vi "ReadLockin_ETH_2median.vi"(0 "Delay (ms)":u32, 1 "Lockin Address":string="1:8", 2 "Integration (ms)":u32=1000, 3 "data storage rate (Hz)":u16(ring)=7 items=[".0625 ", "0.125 ", "0.250 ", "0.500 ", "1 ", "2 ", "4", "8 ", "16 ", "32 ", "64 ", "128", "256", "512"], 5 "error in":errorcluster) -> (6 "R":dbl=0.0024531641755826043, 7 "Theta (radians)":dbl=2.561846938936039, 8 "error out":errorcluster)   [LabVIEW 2023]
uses:
  <vilib>/Analysis/NI_AALBase.lvlib
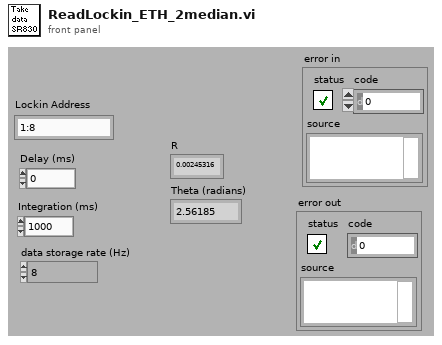
[diagram p1: front panel]
types:
  T1 = cluster{"error":bool, "code":i32, "source":string}
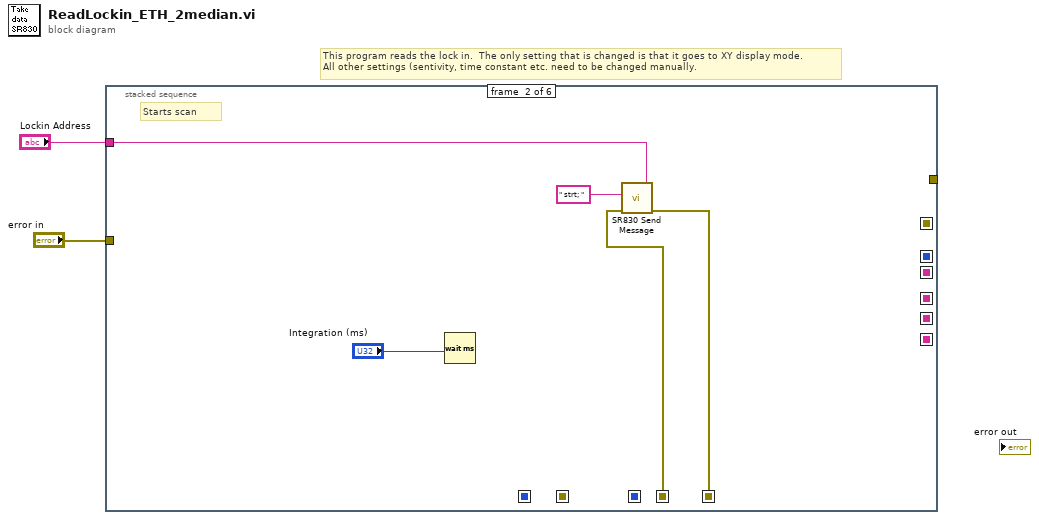
[diagram p0: block diagram]
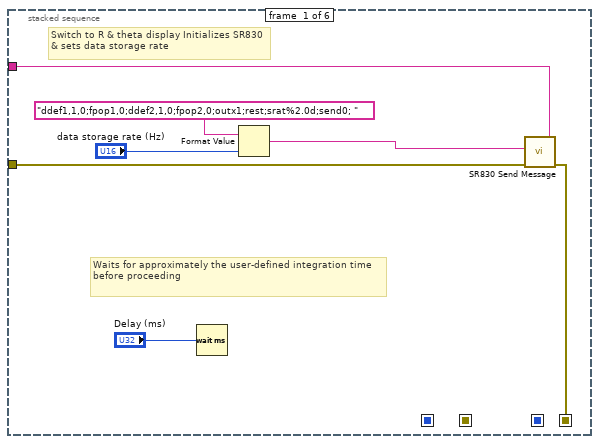
[diagram p2: hidden frame]
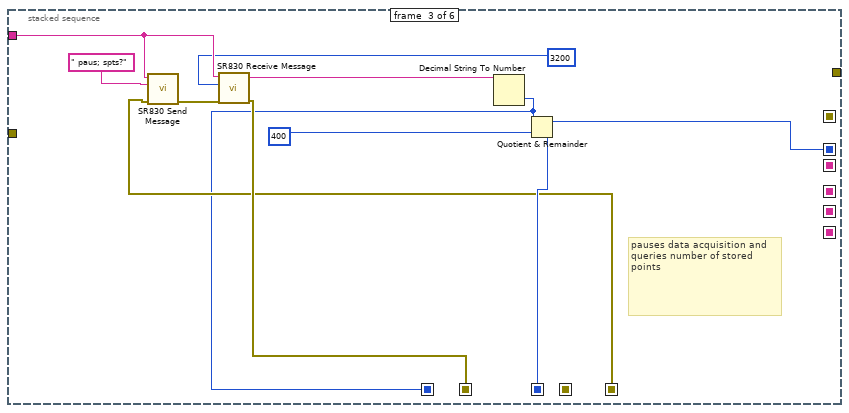
[diagram p3: hidden frame]
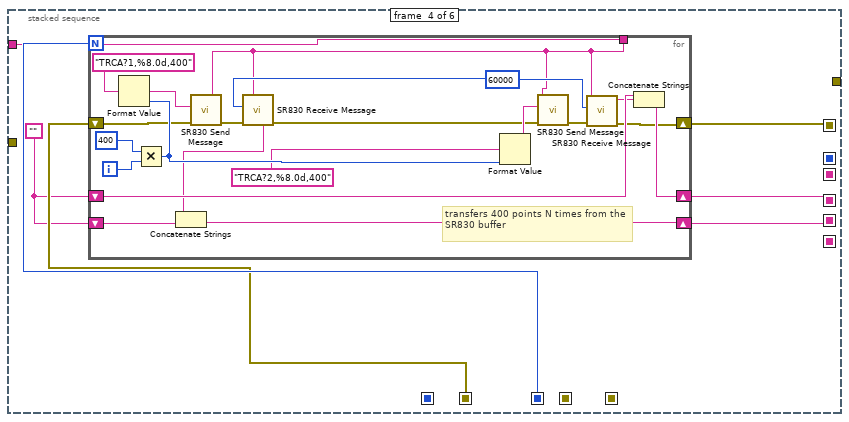
[diagram p4: hidden frame]
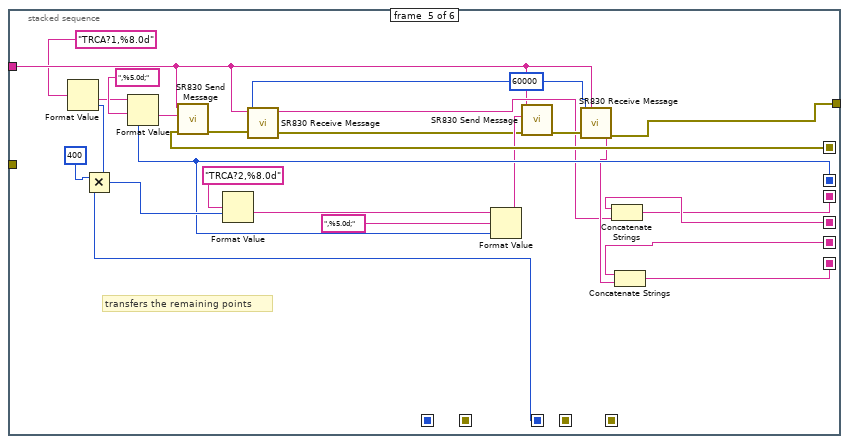
[diagram p5: hidden frame]
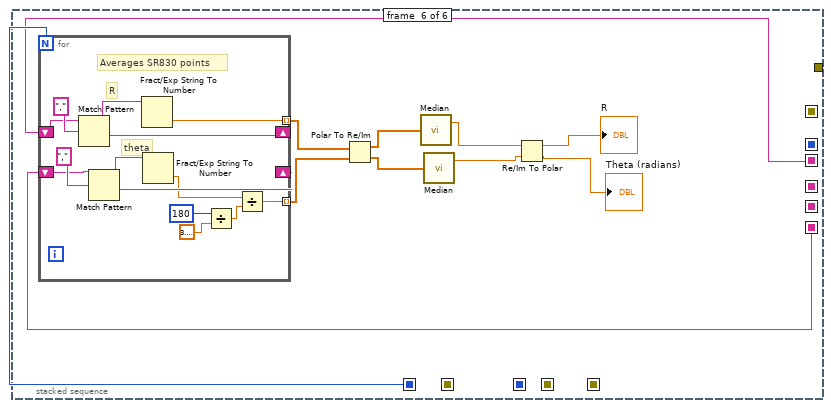
[diagram p6: hidden frame]
diagram:
  # "This program reads the lock in.  The only setting that is changed is that it goes to XY display mode.\nAll other settings (sentivity, time constant etc. need to be changed manually."
  n1 = stacked-sequence {
    seq-local: [w8 _ _ _ _ _] -> [_ w13 _ _ _ _]
    seq-local: [_ _ w24 _ _ _] -> [_ _ _ _ w74 _]
    seq-local: [_ _ w23 _ _ _] -> [_ _ _ w32 w76 _]
    seq-local: [_ _ w17 _ _ _] -> [_ _ _ w30 _ _]
    seq-local: [_ _ _ w28 _ _] -> [_ _ _ _ w71 _]
    seq-local: [_ _ _ w27 _ _] -> [_ _ _ _ w73 _]
    seq-local: [_ _ _ w26 _ _] -> [_ _ _ _ w72 _]
    seq-local: [_ _ w15 _ _ _] -> [_ _ _ _ _ w88]
    seq-local: [_ _ _ _ w54 _] -> [_ _ _ _ _ w86]
    seq-local: [_ _ _ _ w53 _] -> [_ _ _ _ _ w87]
    seq-local: [_ w12 _ _ _ _] -> [_ _ w16 _ _ _]
    tunnel: "error in" -> [w9 _ _ _ _ _]
    tunnel: "Lockin Address" -> [w7 w14 w21 w31 w64 _]
    tunnel: [_ _ _ _ w68 _] -> _
    frame #0 {
      # "Waits for approximately the user-defined integration time before proceeding"
      # "Switch to R & theta display Initializes SR830 & sets data storage rate"
      n2 = Wait (ms)(milliseconds to wait="Delay (ms)") -> ()  [unwired: 1 out]
      n3 = Format Value(format string="ddef1,1,0;fpop1,0;ddef2,1,0;fpop2,0;outx1;rest;srat%2.0d;send0; ", value (0)="data storage rate (Hz)") -> (output string=w4:string)  [unwired: 1 in]
      n4 = call "SR830 Send Message.vi"("address string"=w7, "write buffer"=w4, "error in"=w9) -> ("error out"=w8:T1)  [unwired: 4 in, 2 out]
    }
    frame #1 {
      # "Starts scan"
      n5 = Wait (ms)(milliseconds to wait="Integration (ms)") -> ()  [unwired: 1 out]
      n6 = call "SR830 Send Message.vi"("address string"=w14, "write buffer"=" strt; ", "error in"=w13) -> ("error out"=w12:T1)  [unwired: 4 in, 2 out]
    }
    frame #2 {
      # "pauses data acquisition and queries number of stored points"
      n7 = call "SR830 Send Message.vi"("address string"=w21, "write buffer"=" paus; spts?", "error in"=w16) -> ("error out"=w20:T1)  [unwired: 4 in, 2 out]
      n8 = call "SR830 Receive Message.vi"("address string"=w21, "byte count"=3200, "error in"=w20) -> ("read buffer"=w18:string, "error out"=w17:T1)  [unwired: 4 in, 1 out]
      n9 = Decimal String To Number(string=w18) -> (number=w15:i32)  [unwired: 2 in, 1 out]
      n10 = Quotient & Remainder(x=w15, y=400) -> (x-y*floor(x/y)=w24:i32, floor(x/y)=w23:i32)
    }
    frame #3 {
      w29 = ""
      n11 = for {
        N: w32 -> [_]
        shift-right: [w37] -> w28
        shift-left: w30 -> [w45]
        tunnel: w31 -> [w38]
        shift-right: [w50] -> w26
        shift-left: w29 -> [w49]
        shift-right: [w46] -> w27
        shift-left: w29 -> [w47]
        i -> [w52]
        w39 = 60000
        # "transfers 400 points N times from the SR830 buffer"
        n12 = Multiply(x=400, y=w52) -> (x*y=w48:i32)
        n13 = Format Value(format string="TRCA?1,%8.0d,400", value (0)=w48) -> (output string=w43:string)  [unwired: 1 in]
        n14 = call "SR830 Send Message.vi"("address string"=w38, "write buffer"=w43, "error in"=w45) -> ("error out"=w44:T1)  [unwired: 4 in, 2 out]
        n15 = call "SR830 Receive Message.vi"("address string"=w38, "byte count"=w39, "error in"=w44) -> ("read buffer"=w42:string, "error out"=w40:T1)  [unwired: 4 in, 1 out]
        n16 = Concatenate Strings(w42, w49) -> (w50:string)
        n17 = Format Value(format string="TRCA?2,%8.0d,400", value (0)=w48) -> (output string=w41:string)  [unwired: 1 in]
        n18 = call "SR830 Send Message.vi"("address string"=w38, "write buffer"=w41, "error in"=w40) -> ("error out"=w36:T1)  [unwired: 4 in, 2 out]
        n19 = call "SR830 Receive Message.vi"("address string"=w38, "byte count"=w39, "error in"=w36) -> ("read buffer"=w35:string, "error out"=w37:T1)  [unwired: 4 in, 1 out]
        n20 = Concatenate Strings(w47, w35) -> (w46:string)
      }
    }
    frame #4 {
      w63 = 60000
      # "transfers the remaining points"
      n21 = Multiply(x=400, y=w76) -> (x*y=w75:i32)
      n22 = Format Value(format string="TRCA?1,%8.0d", value (0)=w75) -> (output string=w59:string)  [unwired: 1 in]
      n23 = Format Value(string ("")=w59, format string=",%5.0d;", value (0)=w74) -> (output string=w58:string)
      n24 = call "SR830 Send Message.vi"("address string"=w64, "write buffer"=w58, "error in"=w71) -> ("error out"=w66:T1)  [unwired: 4 in, 2 out]
      n25 = Format Value(format string="TRCA?2,%8.0d", value (0)=w75) -> (output string=w55:string)  [unwired: 1 in]
      n26 = call "SR830 Receive Message.vi"("address string"=w64, "byte count"=w63, "error in"=w66) -> ("read buffer"=w65:string, "error out"=w62:T1)  [unwired: 4 in, 1 out]
      n27 = Format Value(string ("")=w55, format string=",%5.0d;", value (0)=w74) -> (output string=w70:string)
      n28 = call "SR830 Send Message.vi"("address string"=w64, "write buffer"=w70, "error in"=w62) -> ("error out"=w69:T1)  [unwired: 4 in, 2 out]
      n29 = call "SR830 Receive Message.vi"("address string"=w64, "byte count"=w63, "error in"=w69) -> ("read buffer"=w67:string, "error out"=w68:T1)  [unwired: 4 in, 1 out]
      n30 = Concatenate Strings(w73, w65) -> (w54:string)
      n31 = Concatenate Strings(w72, w67) -> (w53:string)
    }
    frame #5 {
      n32 = for {
        N: w88 -> [_]
        shift-right: [w98] -> _
        shift-left: w86 -> [w97]
        shift-right: [w96] -> _
        shift-left: w87 -> [w95]
        tunnel: [w94] -> w85 mode=indexing
        tunnel: [w89] -> w84 mode=indexing
        # "Averages SR830 points"
        # "theta"
        # "R"
        n33 = Match Pattern(string=w97, regular expression=",") -> (before substring=w101:string, after substring=w98:string)  [unwired: 1 in, 2 out]
        n34 = Match Pattern(string=w95, regular expression=",") -> (before substring=w100:string, after substring=w96:string)  [unwired: 1 in, 2 out]
        n35 = Fract/Exp String To Number(string=w101) -> (number=w94:dbl)  [unwired: 3 in, 1 out]
        n36 = Fract/Exp String To Number(string=w100) -> (number=w90:dbl)  [unwired: 3 in, 1 out]
        n37 = Divide(x=180, y=3.141592653589793) -> (x/y=w93:dbl)
        n38 = Divide(x=w90, y=w93) -> (x/y=w89:dbl)
      }
      n39 = Polar To Re/Im(2:w84, 3:w85) -> (0:w81:dbl[], 1:w79:dbl[])
      n40 = call <vilib>:"Median.vi"("X"=w79) -> ("median"=w78:dbl)  [unwired: 1 out]
      n41 = call <vilib>:"Median.vi"("X"=w81) -> ("median"=w80:dbl)  [unwired: 1 out]
      n42 = Re/Im To Polar(2:w80, 3:w78) -> (0:→"Theta (radians)":dbl, 1:→"R":dbl)
    }
  }
